vi "Fill Rectangle.vi"(4 "Error":string, 5 "Rectangle":T1, 6 "Value":u8, 7 "Image":T2={"Image ID"=0, "Channel ID"=-1}) -> (0 "Error":string, 3 "Image":T2={"Image ID"=0, "Channel ID"=-1})   [LabVIEW 2011, in "labvvis.lvlib"]
doc: "Fills a rectangle within Image with Value. For RGBA images, all channels in the pixel are set to Value. Thus, this VI can only set grey pixels.\n\nThis VI is useful to creating rectangular masks."
uses:
  <userlib>/labvvis/labvvis.lvlib
  <userlib>/labvvis/VVIS Image.ctl
  <userlib>/labvvis/Rectangle.ctl
  labvvis.framework
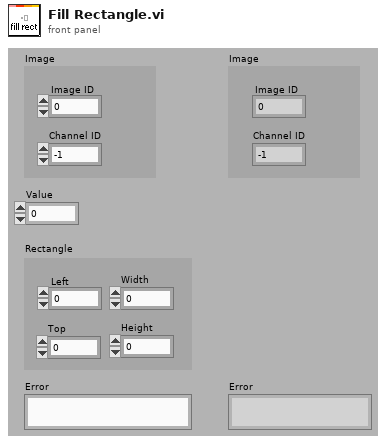
[diagram p1: front panel]
types:
  T1 = typedef "labvvis.lvlib/Rectangle.ctl" = cluster{"Left ":i32, "Top":i32, "Width":i32, "Height":i32}
  T2 = typedef "labvvis.lvlib/VVIS Image.ctl" = cluster{"Image ID":i16, "Channel ID":i16}
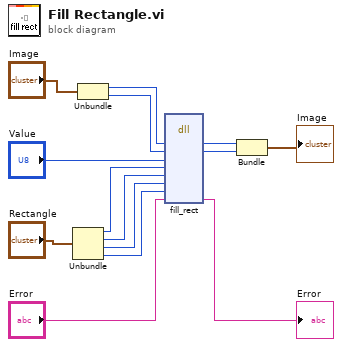
[diagram p0: block diagram]
diagram:
  n1 = Unbundle("Rectangle") -> ("Left"=w9:i32, "Top"=w8:i32, "Width"=w7:i32, "Height"=w6:i32)
  n2 = Unbundle("Image") -> ("Image ID"=w12:i16, "Channel ID"=w11:i16)
  n3 = dll-call lib="labvvis.framework" fn="fill_rect"("out"=w12, "cid"=w11, "value"="Value", "ix"=w9, "iy"=w8, "width"=w7, "height"=w6, "error"="Error") -> ("out"=w3:i16, "cid"=w2:i16, "error"=→"Error":string)  [unwired: 9 in, 2 out]
  n4 = Bundle("out"=w3, "cid"=w2) -> (→"Image":cluster{"out":i16, "cid":i16})  [unwired: 1 in]
